vi "U3 Multiple IO Example Loop 2.vi"() -> ()   [LabVIEW 2021]
panel:
  in  "EIO-CIO States":bool[](array[boolean])=[FALSE, FALSE, FALSE, FALSE, FALSE, FALSE, FALSE, FALSE, FALSE, FALSE, FALSE, FALSE]
  in  "Interval (ms)":u32=500
  in  "stop":bool
  out "AIN3":dbl format="%.6f"
  out "AIN2":dbl format="%.6f"
  out "AIN1":dbl format="%.6f"
  out "AIN0":dbl format="%.6f"
  in  "DAC0":dbl format="%.4f"
  out "Error Message":string
  out "error out":errorcluster
  # "Writes DAC0, writes EIO0-CIO3, and aquires AIN0-AIN3.  Uses USB on the first found U3."
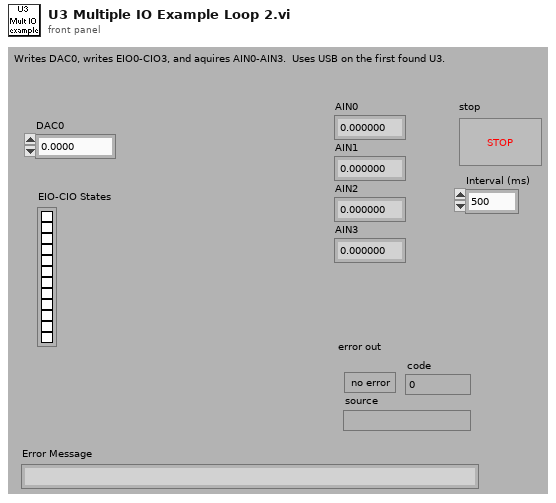
[diagram p1: front panel]
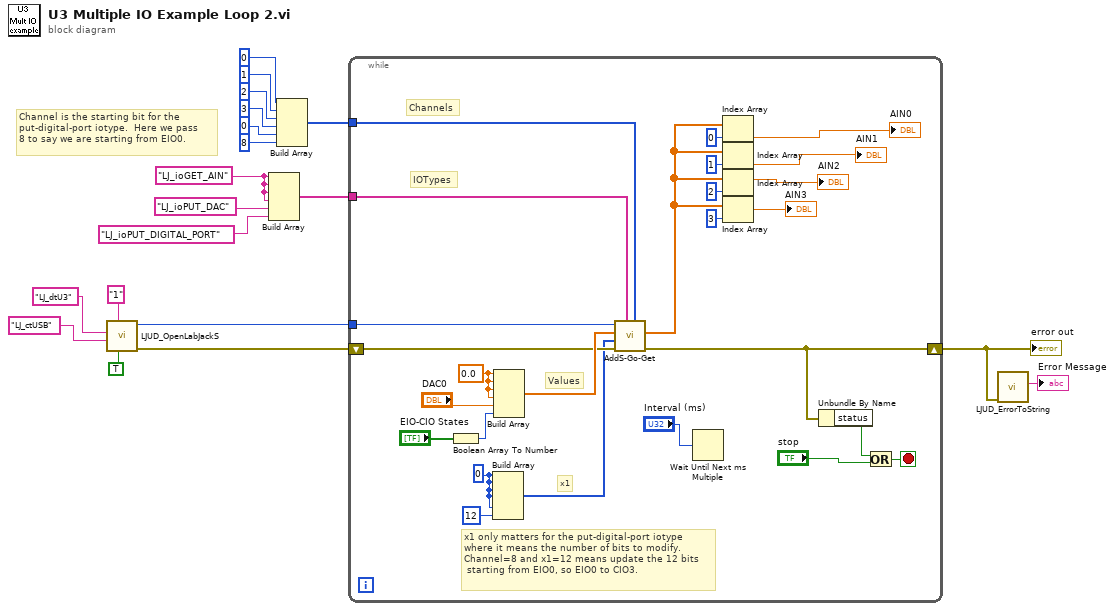
[diagram p0: block diagram]
diagram:
  w18 = "LJ_ioGET_AIN" ("IOType")
  # "Channel is the starting bit for the\nput-digital-port iotype.  Here we pass\n8 to say we are starting from EIO0."
  n1 = call "LJUD_OpenLabJackS.vi"("FirstFound"=TRUE, "Address"="1", "ConnectionType"="LJ_ctUSB", "DeviceType"="LJ_dtU3") -> ("error out"=w3:errorcluster, "Handle"=w4:i32)  [unwired: 5 in, 1 out]
  n2 = Build Array(w18, w18, w18, w18, "LJ_ioPUT_DAC" ("IOType"), "LJ_ioPUT_DIGITAL_PORT" ("IOType")) -> (w17:string[])
  n3 = Build Array(0, 1, 2, 3, 0, 8) -> (w16:i32[])
  n4 = while {
    shift-left: w3 -> [w28]
    shift-right: [w27] -> w5
    tunnel: w4 -> [w32]
    tunnel: w16 -> [w44]
    tunnel: w17 -> [w45]
    stop <- w31 stop-if-true
    w22 = 0 ("Index")
    w43 = 0.0 ("Input Element")
    # "x1 only matters for the put-digital-port iotype\nwhere it means the number of bits to modify.\nChannel=8 and x1=12 means update the 12 bits\n starting from EIO0, so EIO0 to CIO3."
    # "x1"
    # "Values"
    # "IOTypes"
    # "Channels"
    n5 = Boolean Array To Number(Boolean array="EIO-CIO States") -> (number=w23:u32)
    n6 = Build Array(w22, w22, w22, w22, w22, 12 ("element")) -> (w20:i32[])
    n7 = Build Array(w43, w43, w43, w43, "DAC0", w23) -> (w42:dbl[])
    n8 = call "AddS-Go-Get.vi"("Channels"=w44, "IOTypes"=w45, "error in"=w28, "x1"=w20, "Values Write"=w42, "Handle In"=w32) -> ("error out"=w27:errorcluster, "Values Read"=w37:dbl[])  [unwired: 3 in, 1 out]
    n9 = Wait Until Next ms Multiple(millisecond multiple="Interval (ms)") -> ()  [unwired: 1 out]
    n10 = Index Array(array=w37, index=0 ("Index")) -> (element=→"AIN0":dbl)
    n11 = Index Array(array=w37, index=1 ("Index")) -> (element=→"AIN1":dbl)
    n12 = Index Array(array=w37, index=2 ("Index")) -> (element=→"AIN2":dbl)
    n13 = Index Array(array=w37, index=3 ("Index")) -> (element=→"AIN3":dbl)
    n14 = Unbundle By Name(w27) -> ("status"=w29:bool)
    n15 = Or(x=w29, y="stop") -> (x .or. y?=w31:bool)
  }
  "error out" <- w5
  n16 = call "LJUD_ErrorToString.vi"("error in"=w5) -> ("String"=→"Error Message":string)  [unwired: 10 in]
